vi "AssertBool.vi"(11 "Boolean":bool) -> (3 "Boolean":bool)   [LabVIEW 2020, in "OpenLvVision_OpenCv.lvlib"]
uses:
  OpenLvVision_OpenCv.lvlib
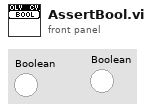
[diagram p1: front panel]
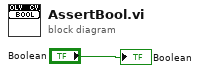
[diagram p0: block diagram]
diagram:
  "Boolean" <- "Boolean"
